vi "CAN Receives FGV.vi"(7 "Action":enum16{"Get", "Put", "Init"}(ring), 8 "length":u8, 9 "data":u8[](array[numeric]), 10 "timestamp":u32, 11 "arb id":u32) -> (3 "Receives":T1(c390))   [LabVIEW 2023]
uses:
  <vilib>/Utility/miscctls.llb/LVMapReplaceAction.ctl
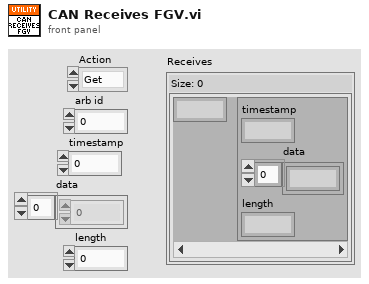
[diagram p1: front panel]
types:
  T1 = map{u32, cluster{"timestamp":u32, "data":u8[], "length":u8}}
  T2 = typedef "LVMapReplaceAction.ctl" = enum32{"Modify Entry only if found", "Add or Modify Entry", "Delete Entry"}
  T3 = cluster{"timestamp":u32, "data":u8[], "length":u8}
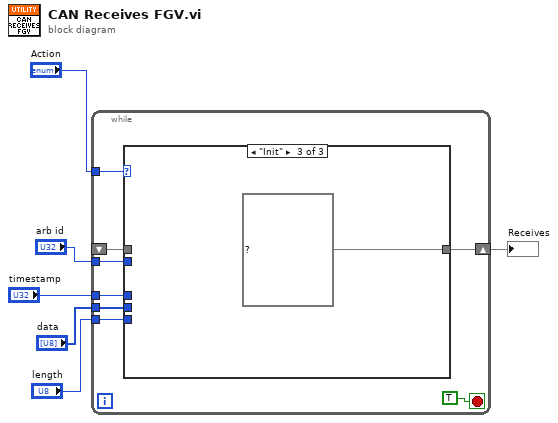
[diagram p0: block diagram]
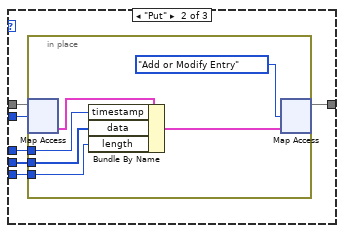
[diagram p3: hidden frame]
diagram:
  n1 = while {
    shift-right: [w12] -> w5
    shift-left: _ -> [w11]
    tunnel: "Action" -> [w13]
    tunnel: "arb id" -> [w10]
    tunnel: "timestamp" -> [w9]
    tunnel: "data" -> [w8]
    tunnel: "length" -> [w7]
    stop <- TRUE stop-if-true
    n2 = case shown="\"Init\"" w13 {
      tunnel: [w15 w19 T1 {} ("Receives")] -> w12
      tunnel: w11 -> [w15 w21 _]
      tunnel: w10 -> [_ w20 _]
      tunnel: w9 -> [_ w18 _]
      tunnel: w8 -> [_ w17 _]
      tunnel: w7 -> [_ w16 _]
      frame "Get", Default {
      }
      frame "Put" {
        n3 = in-place {
          in-place-border: w18 -> [w25]
          in-place-border: w17 -> [w24]
          in-place-border: w16 -> [w23]
          n4 = in-place-map #1(w21, w20) -> (w26:T3)  [unwired: 1 in, 1 out]
          n5 = Bundle By Name(cluster=w26, "timestamp"=w25, "data"=w24, "length"=w23) -> (w27:T3)
          n6 = in-place-map #1(w27, LVMapReplaceAction."Add or Modify Entry" ("action")) -> (w19:T1)  [unwired: 2 out]
        }
      }
      frame "Init" {
      }
    }
  }
  "Receives" <- w5
